vi "queue test.vi"() -> ()   [LabVIEW 2019]
uses:
  Timer Delay/unix time 1s.vi
  Timer Delay/Timers.lvlib
  Database/PostgreSQL2LabVIEW/libpqUtility64/libpqutility64.lvlib
panel:
  out "timed out?":bool
  out "status":bool
  out "ALR_msg":string
  in  "stop":bool
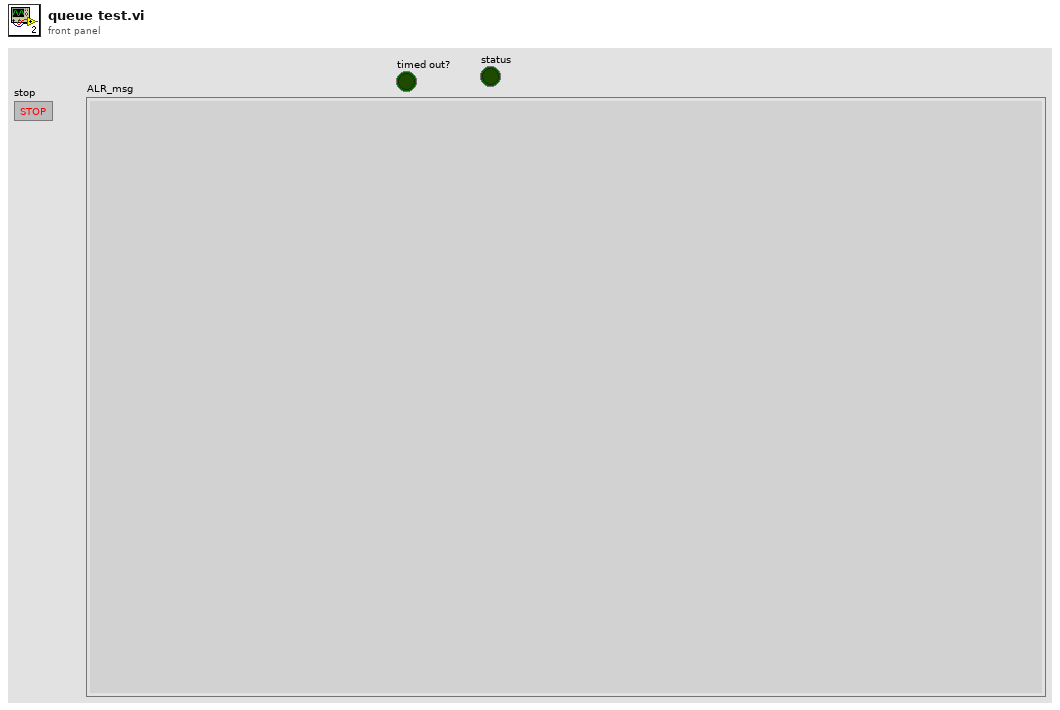
[diagram p1: front panel]
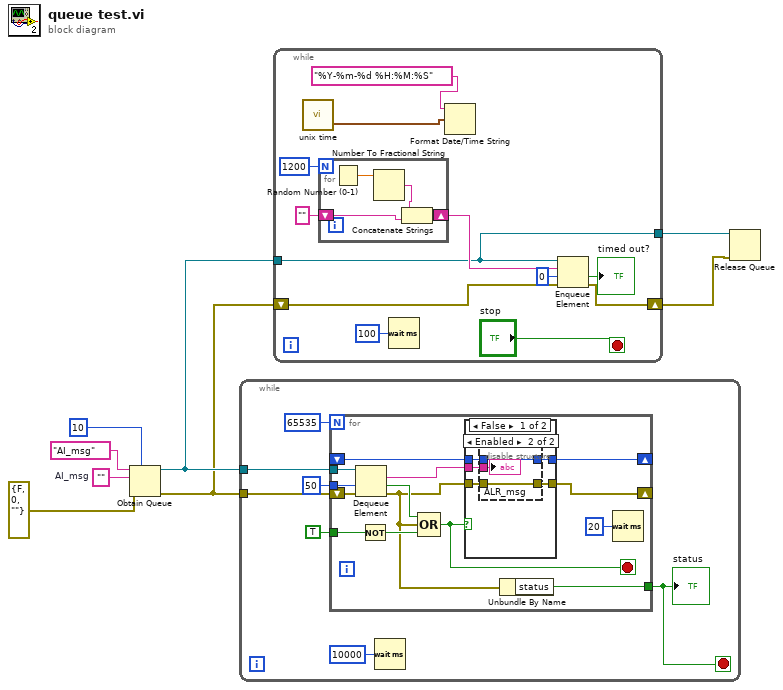
[diagram p0: block diagram]
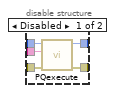
[diagram p2: hidden frame]
diagram:
  w6 = ""  # AI_msg
  n1 = Obtain Queue(max queue size (-1, unlimited)=10, name (unnamed)="AI_msg", element data type=w6, error in (no error)=errorcluster {"status"=FALSE, "code"=0, "source"=""}) -> (queue out=w2:refnum<queue>, error out=w1:errorcluster)  [unwired: 1 in, 1 out]
  n2 = while {
    tunnel: w2 -> [w14]
    tunnel: w1 -> [w13]
    stop <- w9 stop-if-true
    n3 = for {
      N: 65535 -> [_]
      tunnel: w14 -> [w27]
      tunnel: 50 ("read_timeout") -> [w25]
      shift-right: [w24] -> _
      shift-left: _ -> [w28]
      tunnel: TRUE ("write enable") -> [w22]
      shift-right: [w29] -> _
      shift-left: w13 -> [w19]
      tunnel: [w17] -> w9
      stop <- w21 stop-if-true
      n4 = Dequeue Element(queue=w27, timeout in ms (-1)=w25, error in (no error)=w19) -> (element=w26:string, timed out?=w23:bool, error out=w18:errorcluster)  [unwired: 1 out]
      n5 = Not(x=w22) -> (.not. x?=w20:bool)
      n6 = Compound Arithmetic op=OR(w23, w18, w20) -> (w21:bool)
      n7 = case shown="False" w21 {
        tunnel: w18 -> [w34 w44]
        tunnel: w28 -> [w33 w43]
        tunnel: [w30 w44] -> w29
        tunnel: w26 -> [w32 _]
        tunnel: [w31 w43] -> w24
        frame False {
          n8 = disable-structure shown="Enabled" {
            disable-tunnel: w34 -> [w39 w41]
            disable-tunnel: w33 -> [w38 w42]
            disable-tunnel: w32 -> [w37 w40]
            disable-tunnel: [w36 w42] -> w31
            disable-tunnel: [w35 w41] -> w30
            frame Disabled {
              n9 = call "PQexecute.vi"("error in"=w39, "SQL querry"=w37, "conn"=w38) -> ("error out"=w35:errorcluster, "conn_out"=w36:u64)  [unwired: 7 in]
            }
            frame Enabled {
              "ALR_msg" <- w40
            }
          }
        }
        frame True {
        }
      }
      n10 = Unbundle By Name(w18) -> ("status"=w17:bool)
      n11 = Wait (ms)(milliseconds to wait=u32 20) -> ()  [unwired: 1 out]
    }
    "status" <- w9
    n12 = Wait (ms)(milliseconds to wait=u32 10000) -> ()  [unwired: 1 out]
  }
  n13 = while {
    shift-right: [w46] -> w3
    shift-left: w1 -> [w48]
    tunnel: w2 -> [w49]
    tunnel: [w49] -> w4
    stop <- "stop" stop-if-true
    n14 = call-poly "unix time.vi"() -> ("time stamp"=w53:timestamp)  [unwired: 2 in, 1 out]
    n15 = for {
      N: 1200 -> [_]
      shift-right: [w57] -> w50
      shift-left: "" -> [w58]
      n16 = Random Number (0-1)() -> (number: 0 to 1=w60:dbl)
      n17 = Number To Fractional String(number=w60) -> (F-format string=w59:string)  [unwired: 3 in]
      n18 = Concatenate Strings(w59, w58) -> (w57:string)
    }
    n19 = Wait (ms)(milliseconds to wait=u32 100) -> ()  [unwired: 1 out]
    n20 = Format Date/Time String(time format string (%c)="%Y-%m-%d %H:%M:%S", seconds (now)=w53) -> ()  [unwired: 1 in, 1 out]
    n21 = Enqueue Element(queue=w49, element=w50, timeout in ms (-1)=0, error in (no error)=w48) -> (timed out?=→"timed out?":bool, error out=w46:errorcluster)  [unwired: 1 out]
  }
  n22 = Release Queue(queue=w4, error in (no error)=w3) -> ()  [unwired: 1 in, 3 out]
